vi "Calc time of measurement.vi"(1 "Number of Power Line Cycles(50Hz)":dbl=50.0, 2 "2182 -A Params":T1={"Auto Range?"=FALSE, "Man / Selected\n       Range"=enum."10mV", "Enable Digital\n       Filter?"=FALSE, "Filter Type"=enum."Movin", "Filter Count"=1, "      Filter\nWindow (%)"=0.01, "Enable Analog\n       Filter?"=FALSE, "NPLCs"=5} {"NPLCs" min=1 max=10; "Filter\nWindow (%)" min=0.01 max=10.0 step=0.01 format="%.2f"; "Filter Count" min=1 max=100}) -> (0 "Time of one measurement":dbl=7100.0)   [LabVIEW 2013, in "Keithly user program.lvlib"]
uses:
  Keithly user program.lvlib
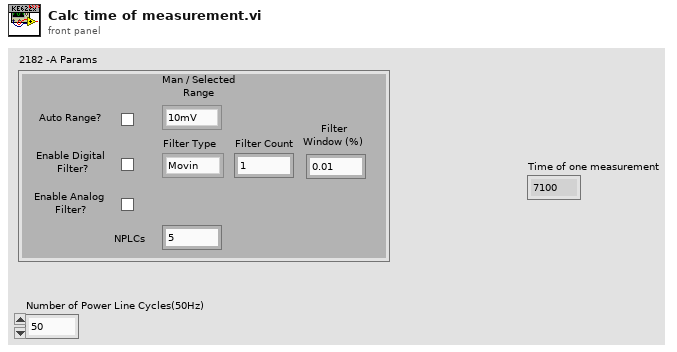
[diagram p1: front panel]
types:
  T1 = cluster{"Auto Range?":bool, "Man / Selected\n       Range":enum16{"10mV", "100mV", "1V", "10V", "100V"}, "Enable Digital\n       Filter?":bool, "Filter Type":enum16{"Movin", "Repeat"}, "Filter Count":u32, "      Filter\nWindow (%)":dbl, "Enable Analog\n       Filter?":bool, "NPLCs":u32}
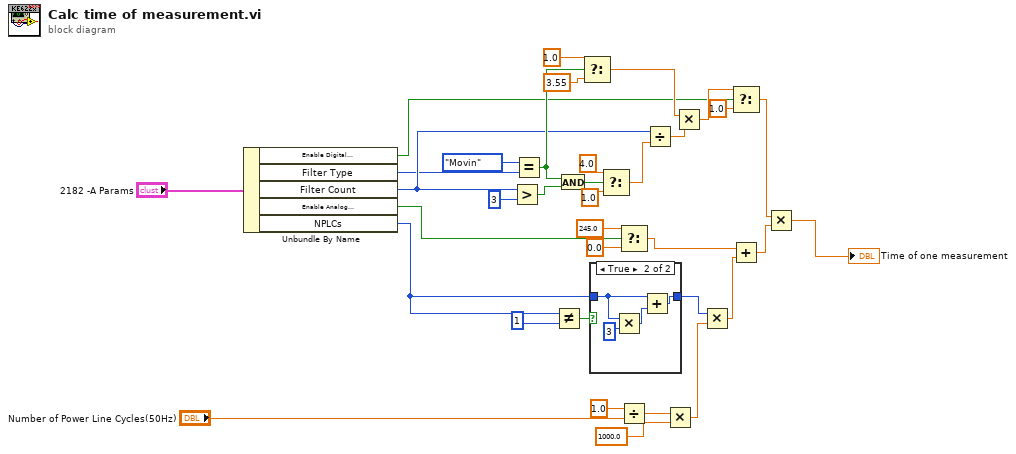
[diagram p0: block diagram]
diagram:
  n1 = Unbundle By Name("2182 -A Params") -> ("Enable Digital\n       Filter?"=w16:bool, "Filter Type"=w22:enum16{"Movin", "Repeat"}, "Filter Count"=w29:u32, "Enable Analog\n       Filter?"=w11:bool, "NPLCs"=w9:u32)
  n2 = Greater?(x=w29, y=u32 3) -> (0:w24:bool)
  n3 = Equal?(x=enum16{"Movin", "Repeat"}."Movin", y=w22) -> (x = y?=w32:bool)
  n4 = Not Equal?(x=w9, y=u32 1) -> (x != y?=w8:bool)
  n5 = And(x=w32, y=w24) -> (x .and. y?=w25:bool)
  n6 = Select(t=1.0 ("f"), s=w32, f=3.55 ("t")) -> (s? t:f=w33:dbl)
  n7 = case shown="True" w8 {
    tunnel: w9 -> [w36 w38]
    tunnel: [w36 w40] -> w10
    frame False {
    }
    frame True {
      n8 = Multiply(x=w38, y=u32 3) -> (x*y=w39:u32)
      n9 = Add(x=w38, y=w39) -> (x+y=w40:u32)
    }
  }
  n10 = Select(t=4.0, s=w25, f=1.0) -> (s? t:f=w28:dbl)
  n11 = Select(t=245.0, s=w11, f=0.0) -> (s? t:f=w14:dbl)
  n12 = Divide(x=1.0, y="Number of Power Line Cycles(50Hz)") -> (x/y=w4:dbl)
  n13 = Divide(x=w29, y=w28) -> (x/y=w30:dbl)
  n14 = Multiply(x=w4, y=1000.0) -> (x*y=w6:dbl)
  n15 = Multiply(x=w33, y=w30) -> (x*y=w31:dbl)
  n16 = Multiply(x=w10, y=w6) -> (x*y=w15:dbl)
  n17 = Select(t=w31, s=w16, f=1.0) -> (s? t:f=w20:dbl)
  n18 = Add(x=w14, y=w15) -> (x+y=w18:dbl)
  n19 = Multiply(x=w20, y=w18) -> (x*y=→"Time of one measurement":dbl)
